vi "Task Manager Message Loop.vi"(8 "error in (no error)":errorcluster caption="错误输入（无错误）", 11 "Message Queues":T1 caption="消息队列") -> (0 "error out":errorcluster caption="错误输出")   [LabVIEW 2015, in "TaskMan.lvlib"]
doc: "该消息循环负责处理硬件数据采集的相关消息。"
uses:
  TaskMan.lvlib
  support/Message Queue/All Message Queues.ctl
  support/Message Queue/Message Cluster.ctl
  TaskMan Configuration.ctl
  TaskSettings.ctl
  TaskMan State.ctl
  support/Message Queue/Enqueue Message (Single).vi
  <vilib>/Utility/error.llb/Error Cluster From Error Code.vi
  <vilib>/ErrorRing/Error Ring.xnode
  support/Message Queue/Message Queue.lvlib
panel:
  out "Message":string caption="消息"
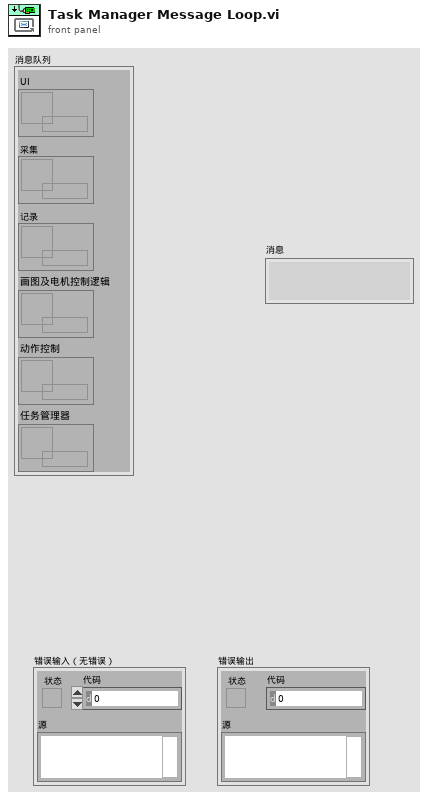
[diagram p1: front panel]
types:
  T1 = typedef "Message Queue.lvlib/All Message Queues.ctl" = cluster{"UI":refnum<queue>, "Acquisition":refnum<queue>, "Logging":refnum<queue>, "plot logic":refnum<queue>, "Action Control":refnum<queue>, "TaskMan":refnum<queue>}
  T2 = typedef "TaskMan.lvlib/TaskMan Configuration.ctl" = cluster{"全自动调阀任务列表":T3}
  T3 = typedef "TaskMan.lvlib/全自动调阀任务列表.ctl" = T4[]
  T4 = typedef "TaskMan.lvlib/TaskSettings.ctl" = cluster{"任务指令":string, "等待时间":dbl}
  T5 = typedef "TaskMan.lvlib/TaskMan State.ctl" = enum16{"Idle", "Acquiring"}
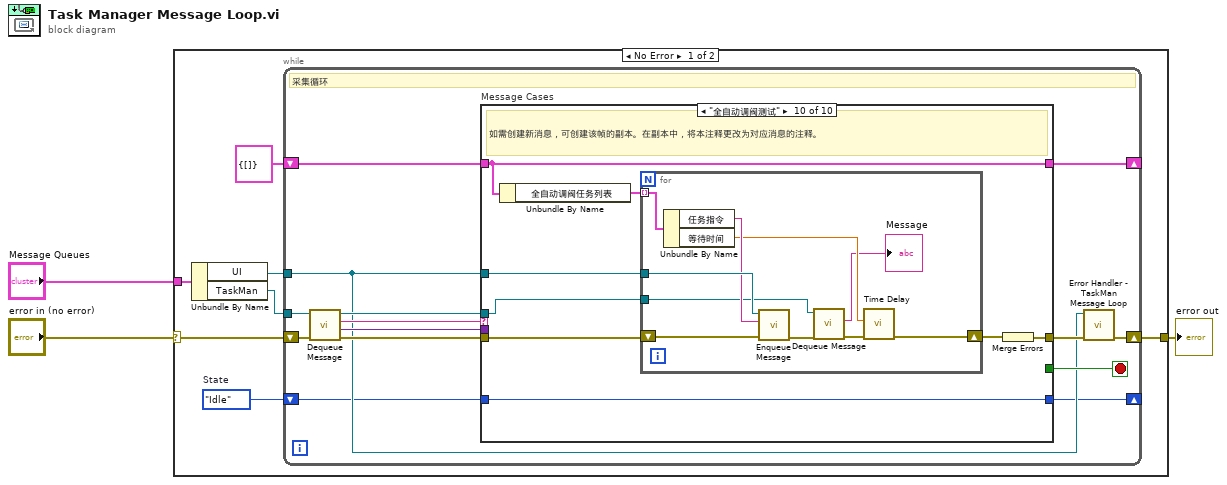
[diagram p0: block diagram]
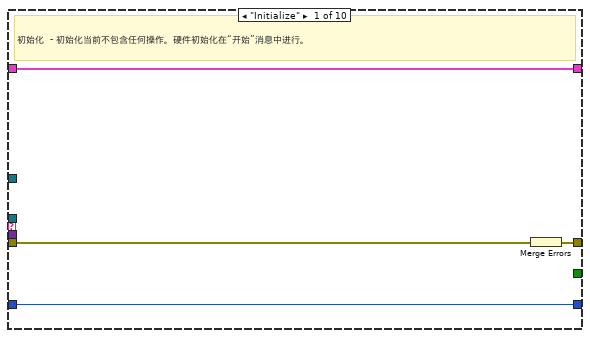
[diagram p2: hidden frame]
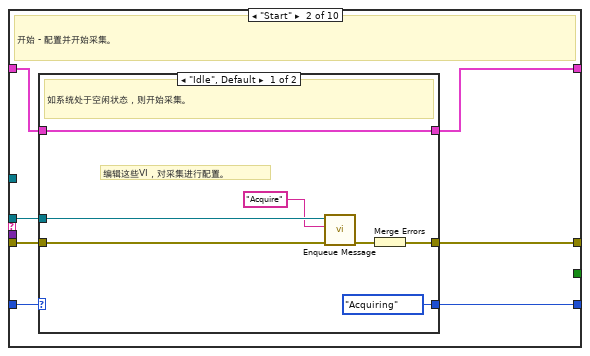
[diagram p3: hidden frame]
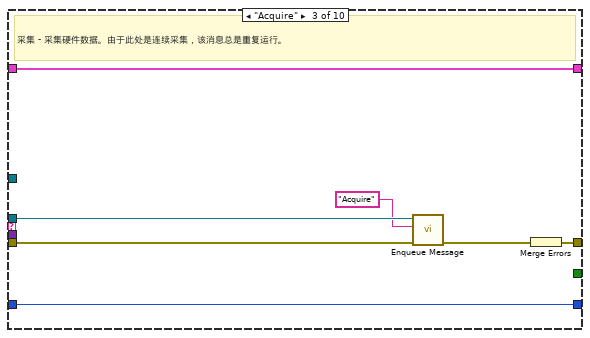
[diagram p5: hidden frame]
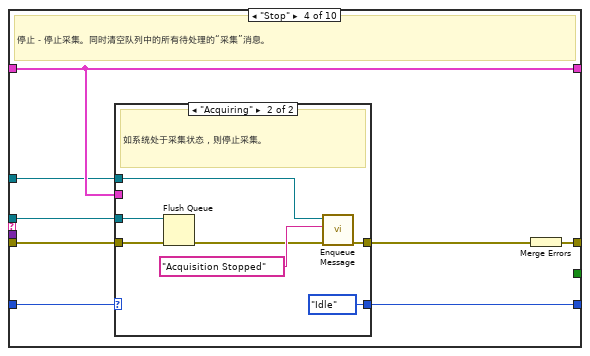
[diagram p6: hidden frame]
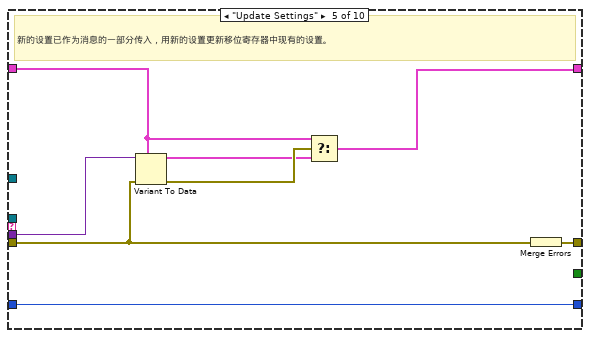
[diagram p8: hidden frame]
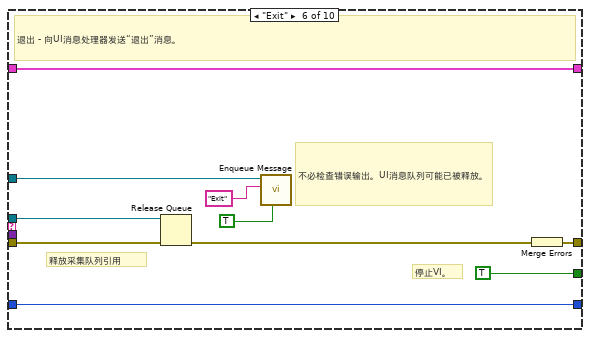
[diagram p9: hidden frame]
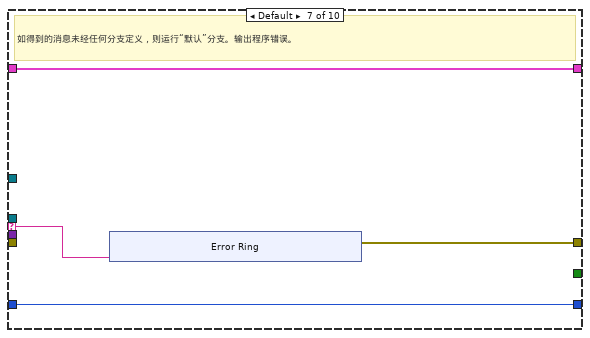
[diagram p10: hidden frame]
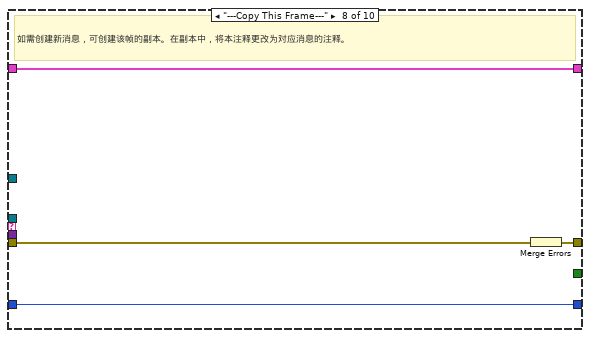
[diagram p11: hidden frame]
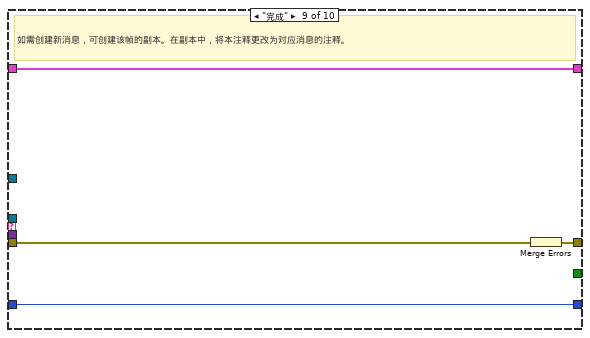
[diagram p12: hidden frame]
diagram:
  n1 = case shown="No Error" "error in (no error)" {
    selector: "error in (no error)" -> [w6 w125]
    tunnel: "Message Queues" -> [w10 _]
    tunnel: [w8 w125] -> w2
    frame No Error {
      w4 = TaskMan_State."Idle"  # State
      n2 = Unbundle By Name(w10) -> ("UI"=w5:refnum<queue>, "TaskMan"=w9:refnum<queue>)
      n3 = while {
        tunnel: w9 -> [w16]
        shift-right: [w23] -> _
        shift-left: T2 {"全自动调阀任务列表"=[]} ("Data Cluster") -> [w24]
        shift-right: [w14] -> w8
        shift-left: w6 -> [w21]
        tunnel: w5 -> [w13]
        shift-right: [w11] -> _
        shift-left: w4 -> [w12]
        stop <- w22 stop-if-true
        # "采集循环"
        n4 = call "Dequeue Message.vi"("error in (no error)"=w21, "Message Queue"=w16) -> ("error out"=w20:errorcluster, "Message Data"=w18:variant, "Message"=w19:string, "dup Message Queue"=w17:refnum<queue>)  [unwired: 6 in]
        n5 = case "Message Cases" shown="\"全自动调阀测试\"" w19 {
          selector: w19 -> [_ _ _ _ _ _ w90 _ _ _]
          tunnel: w17 -> [_ w32 w50 w57 _ w80 _ _ _ w109]
          tunnel: w20 -> [w27 w33 w49 w59 w71 w84 _ w102 w106 w107]
          tunnel: [w28 w35 w52 w60 w77 w86 w89 w100 w104 w114] -> w15
          tunnel: w24 -> [w26 w34 w46 w58 w73 w79 w91 w101 w105 w112]
          tunnel: [w26 w31 w46 w58 w72 w79 w91 w101 w105 w112] -> w23
          tunnel: [_ _ _ _ _ TRUE _ _ _ _] -> w22
          tunnel: w18 -> [_ _ _ _ w76 _ _ _ _ _]
          tunnel: w13 -> [_ _ _ w56 _ w85 _ _ _ w110]
          tunnel: w12 -> [w25 w30 w47 w55 w70 w78 w88 w99 w103 w113]
          tunnel: [w25 w29 w47 w54 w70 w78 w88 w99 w103 w113] -> w11
          frame "Initialize" {
            # "初始化  - 初始化当前不包含任何操作。硬件初始化在“开始”消息中进行。"
            n6 = Merge Errors(w27) -> (w28:errorcluster)
          }
          frame "Start" {
            # "开始 - 配置并开始采集。"
            n7 = case shown="\"Idle\", Default" w30 {
              selector: w30 -> [_ w43]
              tunnel: [w42 w45] -> w35
              tunnel: w34 -> [w36 w44]
              tunnel: w33 -> [w41 w45]
              tunnel: w32 -> [w39 _]
              tunnel: [w36 w44] -> w31
              tunnel: [TaskMan_State."Acquiring" ("State") w43] -> w29
              frame "Idle", Default {
                # "编辑这些VI，对采集进行配置。"
                # "如系统处于空闲状态，则开始采集。"
                n8 = call-poly "Enqueue Message.vi"("error in (no error)"=w41, "Message"="Acquire", "Message Queue"=w39) -> ("error out"=w40:errorcluster)  [unwired: 7 in, 1 out]
                n9 = Merge Errors(w40) -> (w42:errorcluster)
              }
              frame "Acquiring" {
                # "系统已开始采集。忽略“开始”消息。"
              }
            }
          }
          frame "Acquire" {
            # "采集 - 采集硬件数据。由于此处是连续采集，该消息总是重复运行。"
            n10 = call-poly "Enqueue Message.vi"("error in (no error)"=w49, "Message"="Acquire", "Message Queue"=w50) -> ("error out"=w51:errorcluster)  [unwired: 7 in, 1 out]
            n11 = Merge Errors(w51) -> (w52:errorcluster)
          }
          frame "Stop" {
            # "停止－停止采集。同时清空队列中的所有待处理的“采集”消息。"
            n12 = case shown="\"Acquiring\"" w55 {
              selector: w55 -> [w62 _]
              tunnel: w59 -> [w61 w69]
              tunnel: w58 -> [_ _]
              tunnel: w57 -> [_ w68]
              tunnel: w56 -> [_ w67]
              tunnel: [w62 TaskMan_State."Idle" ("State")] -> w54
              tunnel: [w61 w66] -> w53
              frame "Idle", Default {
                # "系统已处于空闲状态。忽略“停止”消息。"
              }
              frame "Acquiring" {
                # "如系统处于采集状态，则停止采集。"
                n13 = Flush Queue(queue=w68, error in (no error)=w69) -> (error out=w63:errorcluster)  [unwired: 2 out]
                n14 = call-poly "Enqueue Message.vi"("error in (no error)"=w63, "Message"="Acquisition Stopped", "Message Queue"=w67) -> ("error out"=w66:errorcluster)  [unwired: 7 in, 1 out]
              }
            }
            n15 = Merge Errors(w53) -> (w60:errorcluster)
          }
          frame "Update Settings" {
            # "新的设置已作为消息的一部分传入，用新的设置更新移位寄存器中现有的设置。"
            n16 = Variant To Data(error in=w71, type=w73, Variant=w76) -> (data=w74:T2, error out=w75:errorcluster)
            n17 = Select(t=w73, s=w75, f=w74) -> (s? t:f=w72:T2)
            n18 = Merge Errors(w71) -> (w77:errorcluster)
          }
          frame "Exit" {
            # "不必检查错误输出。UI消息队列可能已被释放。"
            # "释放采集队列引用"
            # "停止VI。"
            # "退出 - 向UI消息处理器发送“退出”消息。"
            n19 = Release Queue(queue=w80, error in (no error)=w84) -> (error out=w81:errorcluster)  [unwired: 1 in, 2 out]
            n20 = call-poly "Enqueue Message.vi"("Priority Message? (F)"=TRUE, "Message"="Exit", "Message Queue"=w85) -> ()  [unwired: 7 in, 2 out]
            n21 = Merge Errors(w81) -> (w86:errorcluster)
          }
          frame Default {
            # "如得到的消息未经任何分支定义，则运行“默认”分支。输出程序错误。"
            n22 = xnode "Error Ring"("parameter 0"=w90) -> ("error out"=w89:errorcluster)
          }
          frame "---Copy This Frame---" {
            # "如需创建新消息，可创建该帧的副本。在副本中，将本注释更改为对应消息的注释。"
            n23 = Merge Errors(w102) -> (w100:errorcluster)
          }
          frame "完成" {
            # "如需创建新消息，可创建该帧的副本。在副本中，将本注释更改为对应消息的注释。"
            n24 = Merge Errors(w106) -> (w104:errorcluster)
          }
          frame "全自动调阀测试" {
            # "如需创建新消息，可创建该帧的副本。在副本中，将本注释更改为对应消息的注释。"
            n25 = Unbundle By Name(w112) -> ("全自动调阀任务列表"=w111:T3)
            n26 = for {
              tunnel: w111 -> [w124] mode=indexing
              tunnel: w110 -> [w123]
              tunnel: w109 -> [w120]
              shift-right: [w117] -> w108
              shift-left: w107 -> [w116]
              n27 = Unbundle By Name(w124) -> ("任务指令"=w122:string, "等待时间"=w118:dbl)
              n28 = call-poly "Enqueue Message.vi"("error in (no error)"=w116, "Message"=w122, "Message Queue"=w123) -> ("error out"=w121:errorcluster)  [unwired: 7 in, 1 out]
              n29 = call "Dequeue Message.vi"("error in (no error)"=w121, "Message Queue"=w120) -> ("error out"=w119:errorcluster, "Message"=→"Message":string)  [unwired: 6 in, 2 out]
              n30 = call "Time Delay"("error in (no error)"=w119, "Delay Time (s)"=w118) -> ("error out"=w117:errorcluster)  [unwired: 9 in]
            }
            n31 = Merge Errors(w108) -> (w114:errorcluster)
          }
        }
        n32 = call "Error Handler - TaskMan Message Loop.vi"("error in (no error)"=w15, "Message Queue"=w13) -> ("dup error in"=w14:errorcluster)  [unwired: 8 in, 1 out]
      }
    }
    frame Error {
    }
  }
  "error out" <- w2
